vi "Get_DI.vi"(8 "error in (no error)":errorcluster, 10 "PIN Number":i8, 11 "DI_DO in":refnum<class "DI_DO.lvclass">) -> (0 "error out":errorcluster, 2 "STATUS":string, 3 "DI_DO out":refnum<class "DI_DO.lvclass">)   [LabVIEW 2023, in "Driver_DI_DO.lvlib" / "DI_DO.lvclass"]
uses:
  DI_DO.lvclass
  DI_DO.lvclass/DI_DO.ctl
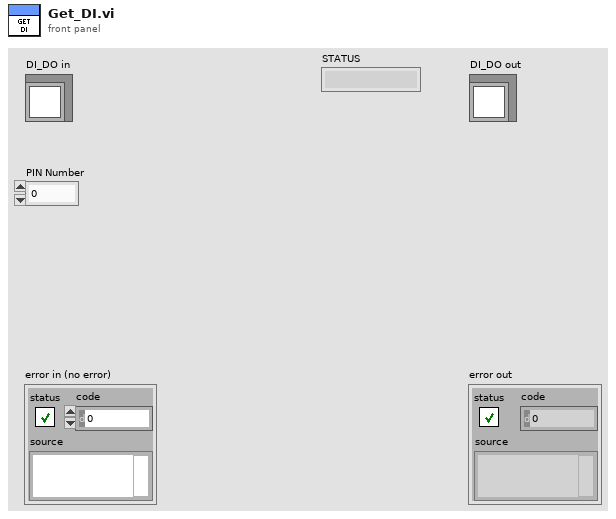
[diagram p1: front panel]
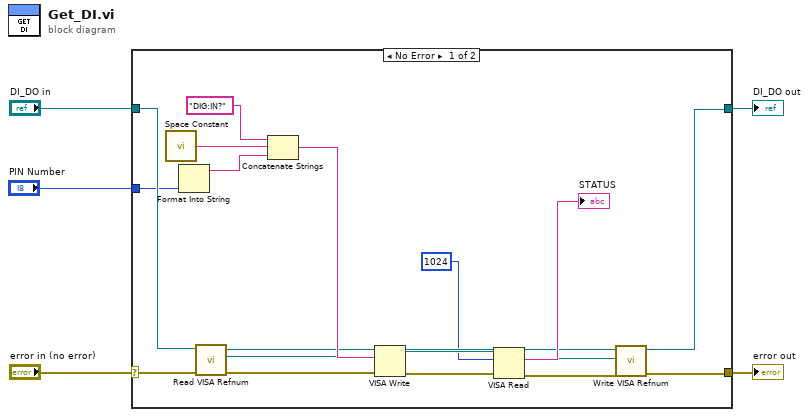
[diagram p0: block diagram]
diagram:
  n1 = case shown="No Error" "error in (no error)" {
    selector: "error in (no error)" -> [w10 w25]
    tunnel: [w7 w25] -> w4
    tunnel: [w6 w24] -> w2
    tunnel: "DI_DO in" -> [w9 w24]
    tunnel: "PIN Number" -> [w8 _]
    frame No Error {
      n2 = call <vilib>:"Space Constant.vi"() -> ("String"=w21:string)
      n3 = Format Into String(w8) -> (resulting string=w22:string)  [unwired: 3 in, 1 out]
      n4 = call-dynamic "Read VISA Refnum.vi"("error in (no error)"=w10, "Driver in"=w9) -> ("error out"=w16:errorcluster, "VISA Refnum"=w15:refnum<visa-resource-name>, "Driver out"=w18:refnum<class "DI_DO.lvclass">)  [unwired: 7 in]
      n5 = Concatenate Strings("DIG:IN?" ("string"), w21, w22) -> (w23:string)
      n6 = VISA Write(VISA resource name=w15, write buffer=w23, error in (no error)=w16) -> (VISA resource name out=w14:refnum<visa-resource-name>, error out=w13:errorcluster)  [unwired: 1 out]
      n7 = VISA Read(VISA resource name=w14, byte count=u32 1024, error in (no error)=w13) -> (VISA resource name out=w19:refnum<visa-resource-name>, read buffer=→"STATUS":string, error out=w17:errorcluster)  [unwired: 1 out]
      n8 = call-dynamic "Write VISA Refnum.vi"("error in (no error)"=w17, "VISA Refnum"=w19, "Driver in"=w18) -> ("error out"=w7:errorcluster, "Driver out"=w6:refnum<class "DI_DO.lvclass">)  [unwired: 7 in]
    }
    frame Error {
    }
  }
  "error out" <- w4
  "DI_DO out" <- w2
